vi "TMxFlexTestSuite.vi"() -> ()   [LabVIEW 2015]
uses:
  State Machine/State Machine.lvlib
panel:
  out "Logs":string
  in  "TEST LIST":i32(listbox)=-1
  in  "Launch Test":bool
  in  "Stop":bool
  # "Overview: TMxFlexTestSuite is to provide a consitent way to invoke every  TMxFlex test package.\nRequirements: Windows\nInstructions:\n1) Select a test package in the provided test list.\n2) Click LAUNCH button to lauch the selected test package.\n3) Click STOP button to terminate TMxFlexTestSuite."
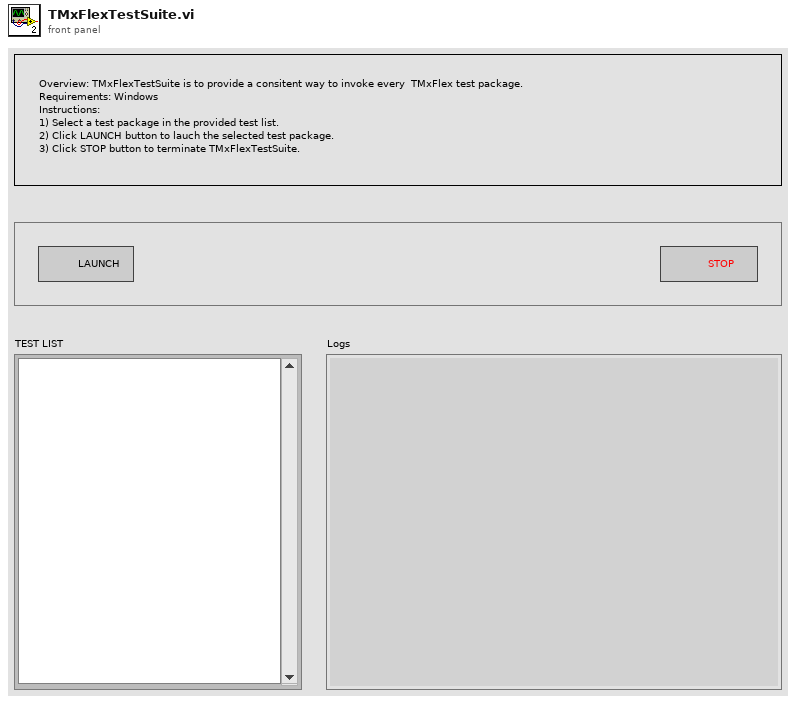
[diagram p1: front panel]
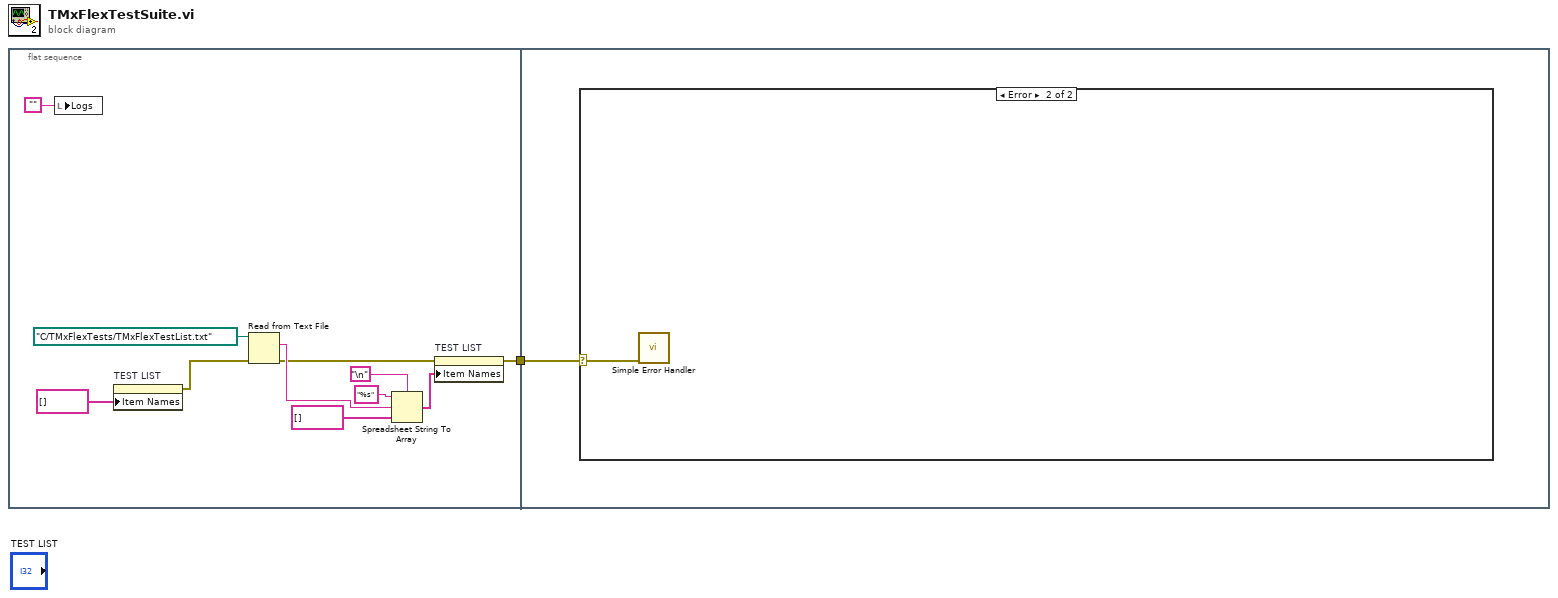
[diagram p0: block diagram]
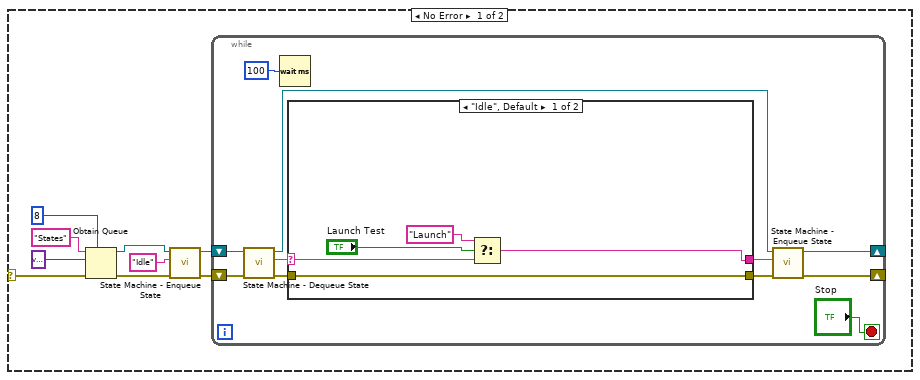
[diagram p2: hidden frame]
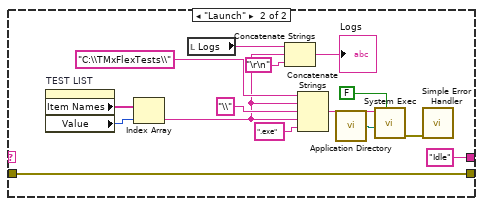
[diagram p3: hidden frame]
diagram:
  n1 = flat-sequence {
    tunnel: [w6] -> w1
    tunnel: w1 -> [w13]
    frame #0 {
      n2 = local write "Logs"("") -> ()
      n3 = property on="TEST LIST" class="LstBox (strict)"("Item Names"=string[] []) -> (error out=w2:errorcluster)  [unwired: 2 in, 1 out]
      n4 = Read from Text File(file (use dialog)=path "C:/TMxFlexTests/TMxFlexTestList.txt", error in=w2) -> (text=w11:string, error out=w7:errorcluster)  [unwired: 2 in, 2 out]
      n5 = Spreadsheet String To Array(delimiter (Tab)="\n", format string="%s", spreadsheet string=w11, array type (2D Dbl)=string[] []) -> (array=w8:string[])
      n6 = property on="TEST LIST" class="LstBox (strict)"(error in=w7, "Item Names"=w8) -> (error out=w6:errorcluster)  [unwired: 1 in, 1 out]
    }
    frame #1 {
      n7 = case shown="Error" w13 {
        selector: w13 -> [w14 w54]
        frame No Error {
          n8 = Obtain Queue(max queue size (-1, unlimited)=8, name (unnamed)="States", element data type=variant, error in (no error)=w14) -> (queue out=w18:refnum<queue>, error out=w19:errorcluster)  [unwired: 1 in, 1 out]
          n9 = call "State Machine - Enqueue State.vi"("error in (no error)"=w19, "State"="Idle", "Queue In"=w18) -> ("error out"=w22:errorcluster, "Queue Out"=w21:refnum<queue>)  [unwired: 7 in]
          n10 = while {
            shift-right: [w25] -> _
            shift-left: w21 -> [w32]
            shift-right: [w27] -> _
            shift-left: w22 -> [w31]
            stop <- "Stop" stop-if-true
            n11 = call "State Machine - Dequeue State.vi"("error in (no error)"=w31, "Queue In"=w32) -> ("error out"=w29:errorcluster, "State"=w33:string, "Queue Out"=w26:refnum<queue>)  [unwired: 5 in, 2 out]
            n12 = Wait (ms)(milliseconds to wait=u32 100) -> ()  [unwired: 1 out]
            n13 = case shown="\"Idle\", Default" w33 {
              selector: w33 -> [w37 _]
              tunnel: [w38 w43] -> w23
              tunnel: w29 -> [w38 w43]
              tunnel: [w34 "Idle"] -> w28
              frame "Idle", Default {
                n14 = Select(t="Launch", s="Launch Test", f=w37) -> (s? t:f=w34:string)
              }
              frame "Launch" {
                n15 = property on="TEST LIST" class="LstBox (strict)"() -> ("Item Names"=w51:string[], "Value"=w52:i32)  [unwired: 2 in, 2 out]
                n16 = Index Array(array=w51, index=w52) -> (element=w40:string)
                n17 = local read "Logs"() -> (w39:string)
                n18 = Concatenate Strings(w39, w40, "\r\n") -> (→"Logs":string)
                n19 = Concatenate Strings("C:\\TMxFlexTests\\" ("string"), w40, "\\" ("string"), w40, ".exe" ("string")) -> (w44:string)
                n20 = call <vilib>:"Application Directory.vi"() -> ("Application Directory"=w48:path)
                n21 = call <vilib>:"System Exec.vi"("wait until completion? (T)"=FALSE, "working directory"=w48, "command line"=w44) -> ("error out"=w42:errorcluster)  [unwired: 5 in, 3 out]
                n22 = call <vilib>:"Simple Error Handler.vi"("error in (no error)"=w42) -> ()  [unwired: 4 in, 5 out]
              }
            }
            n23 = call "State Machine - Enqueue State.vi"("error in (no error)"=w23, "State"=w28, "Queue In"=w26) -> ("error out"=w27:errorcluster, "Queue Out"=w25:refnum<queue>)  [unwired: 7 in]
          }
        }
        frame Error {
          n24 = call <vilib>:"Simple Error Handler.vi"("error in (no error)"=w54) -> ()  [unwired: 4 in, 5 out]
        }
      }
    }
  }
